vi "Write Gui_TestCtrl.vi"(8 "error in (no error)":errorcluster, 10 "Gui_TestCtrl":T1, 11 "GUI_Handler_Seq in":refnum<class "GUI_Handler_Seq.lvclass">) -> (0 "error out":errorcluster, 3 "GUI_Handler_Seq out":refnum<class "GUI_Handler_Seq.lvclass">)   [LabVIEW 2017, in "GUI_Handler_Seq.lvclass"]
uses:
  GUI_Handler_Seq.lvclass
  GUI_Handler_Seq.lvclass/GUI_Handler_Seq.ctl
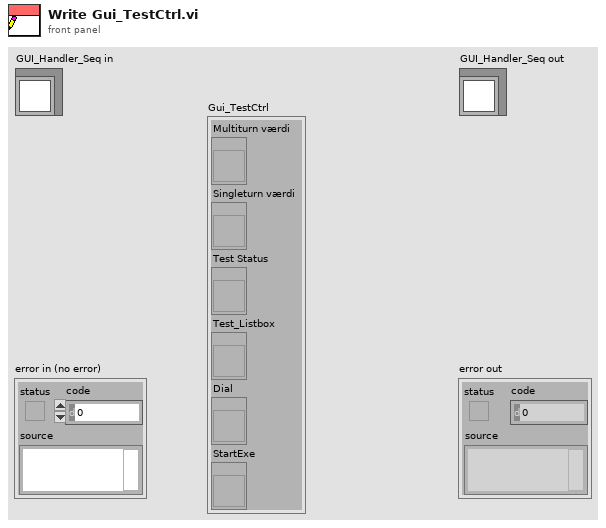
[diagram p1: front panel]
types:
  T1 = cluster{"Multiturn værdi":refnum<vi>, "Singleturn værdi":refnum<vi>, "Test Status":refnum<vi>, "Test_Listbox":refnum<vi>, "Dial":refnum<vi>, "StartExe":refnum<vi>}
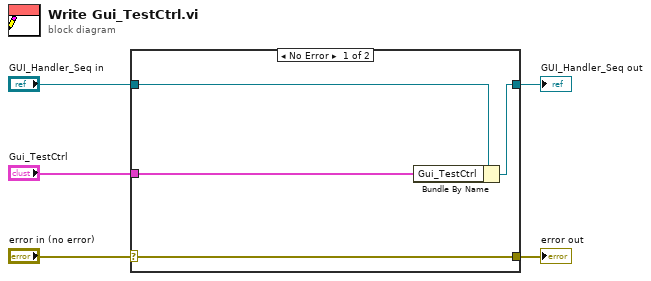
[diagram p0: block diagram]
diagram:
  n1 = case shown="No Error" "error in (no error)" {
    selector: "error in (no error)" -> [w9 w10]
    tunnel: [w9 w10] -> w4
    tunnel: [w7 w11] -> w2
    tunnel: "GUI_Handler_Seq in" -> [w8 w11]
    tunnel: "Gui_TestCtrl" -> [w6 _]
    frame No Error {
      n2 = Bundle By Name(cluster=w8, "Gui_TestCtrl"=w6) -> (w7:refnum<class "GUI_Handler_Seq.lvclass">)
    }
    frame Error {
    }
  }
  "error out" <- w4
  "GUI_Handler_Seq out" <- w2
